vi "UsrProfiles-Users shortcut activ handler.vi"(10 "Users ListBox MenuRef":refnum<k9>, 11 "Users ListBox ref":refnum<vi>) -> ()   [LabVIEW 2017]
panel:
  in  "error in":errorcluster
  out "error out":errorcluster
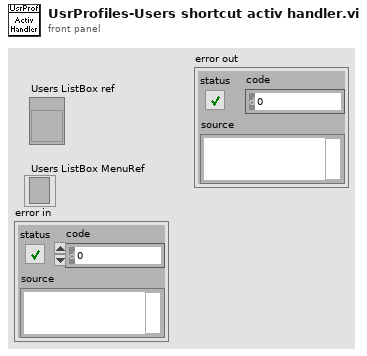
[diagram p1: front panel]
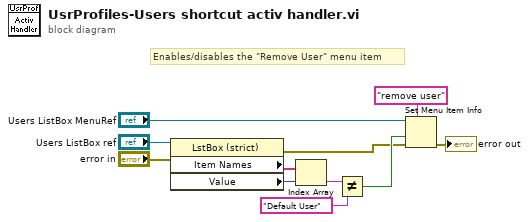
[diagram p0: block diagram]
diagram:
  # "Enables/disables the \"Remove User\" menu item"
  n1 = property on="Property Node" class="LstBox (strict)"(reference="Users ListBox ref", error in="error in") -> (error out=w4:errorcluster, "Item Names"=w8:string[], "Value"=w9:i32)  [unwired: 1 out]
  n2 = Index Array(array=w8, index=w9) -> (element=w10:string)
  n3 = Not Equal?(x=w10, y="Default User") -> (x != y?=w5:bool)
  n4 = Set Menu Item Info(7:"remove user" ("item name"), 8:w4, 9:w5, 11:"Users ListBox MenuRef") -> (0:→"error out":errorcluster)  [unwired: 3 in, 1 out]
